vi "AngularCalib.vi"(7 "B [T]":dbl, 10 "Clibration":T13={"cam 0"={"incident ANGLE COMPENSATION"=[], "dp/B [MeV/C/B]"=[], "charge compensation"=[], "Momentum [MeV/C]"=[], "energyDependence Input"=[], "pixel angle (y)"=[], "dp [MeV/C/] "=[], "angle 2Dfor spectrumj"=[], "dp [MeV/C] 2D"=[], "charge compensation 2D"=[], "Screen&Camera 2"={"Screen Orientation"="Regular", "Screen angle"="Flat", "Lens"=enum."FL1-f8x08", "Calibration (mm/pix)"=1.0}, "ROI info"={"npix-X"=0, "npix-Y"=0, "Left [pix]"=0.0, "Top [pix]"=0.0}, "Y 2D full angle"=[], "calib pixel"={"y1(pixel)"=[], "y2(pixel)"=[], "dp/B [MeV/C/B] (pixel)"=[], "energyDependence Input(pixel)"=[], "bending angle [deg](pixel)"=[], "total path(pixel)"=[], "pixel angle (y)(pixel)"=[], "energy dependence (pixel)"=[], "charge compensation (pixel)"=[], "Momentum [MeV/C](pixel)"=[], "angular compensation(pixel)"=[]}, "2D"={"dp"=[], "chargeCompensation"=[], "angle"=[], "Momentum"=[]}, "UserROI"={"Width"=0.0, "Hight"=0.0, "OffsetX"=0.0, "OffsetY"=0.0}, "final"={"X"=[], "xi"=[], "delta momentum"=0.0, "Y"=[], "yi"=[], "angle (Y)"=[], "delta angle"=0.0, "scale delta angle"=0.0, "intraX"=0.0, "intraY"=0.0, "mask"=[]}, "B[T]"=0.0, "index"=0.0}, "cam 1"={"incident ANGLE COMPENSATION"=[], "dp/B [MeV/C/B]"=[], "charge compensation"=[], "Momentum [MeV/C]"=[], "energyDependence Input"=[], "pixel angle (y)"=[], "dp [MeV/C/] "=[], "angle 2Dfor spectrumj"=[], "dp [MeV/C] 2D"=[], "charge compensation 2D"=[], "Screen&Camera 2"={"Screen Orientation"="Regular", "Screen angle"="Flat", "Lens"=enum."FL1-f8x08", "Calibration (mm/pix)"=1.0}, "ROI info"={"npix-X"=0, "npix-Y"=0, "Left [pix]"=0.0, "Top [pix]"=0.0}, "Y 2D full angle"=[], "calib pixel"={"y1(pixel)"=[], "y2(pixel)"=[], "dp/B [MeV/C/B] (pixel)"=[], "energyDependence Input(pixel)"=[], "bending angle [deg](pixel)"=[], "total path(pixel)"=[], "pixel angle (y)(pixel)"=[], "energy dependence (pixel)"=[], "charge compensation (pixel)"=[], "Momentum [MeV/C](pixel)"=[], "angular compensation(pixel)"=[]}, "2D"={"dp"=[], "chargeCompensation"=[], "angle"=[], "Momentum"=[]}, "UserROI"={"Width"=0.0, "Hight"=0.0, "OffsetX"=0.0, "OffsetY"=0.0}, "final"={"X"=[], "xi"=[], "delta momentum"=0.0, "Y"=[], "yi"=[], "angle (Y)"=[], "delta angle"=0.0, "scale delta angle"=0.0, "intraX"=0.0, "intraY"=0.0, "mask"=[]}, "B[T]"=0.0, "index"=0.0}, "cam 2"={"incident ANGLE COMPENSATION"=[], "dp/B [MeV/C/B]"=[], "charge compensation"=[], "Momentum [MeV/C]"=[], "energyDependence Input"=[], "pixel angle (y)"=[], "dp [MeV/C/] "=[], "angle 2Dfor spectrumj"=[], "dp [MeV/C] 2D"=[], "charge compensation 2D"=[], "Screen&Camera 2"={"Screen Orientation"="Regular", "Screen angle"="Flat", "Lens"=enum."FL1-f8x08", "Calibration (mm/pix)"=1.0}, "ROI info"={"npix-X"=0, "npix-Y"=0, "Left [pix]"=0.0, "Top [pix]"=0.0}, "Y 2D full angle"=[], "calib pixel"={"y1(pixel)"=[], "y2(pixel)"=[], "dp/B [MeV/C/B] (pixel)"=[], "energyDependence Input(pixel)"=[], "bending angle [deg](pixel)"=[], "total path(pixel)"=[], "pixel angle (y)(pixel)"=[], "energy dependence (pixel)"=[], "charge compensation (pixel)"=[], "Momentum [MeV/C](pixel)"=[], "angular compensation(pixel)"=[]}, "2D"={"dp"=[], "chargeCompensation"=[], "angle"=[], "Momentum"=[]}, "UserROI"={"Width"=0.0, "Hight"=0.0, "OffsetX"=0.0, "OffsetY"=0.0}, "final"={"X"=[], "xi"=[], "delta momentum"=0.0, "Y"=[], "yi"=[], "angle (Y)"=[], "delta angle"=0.0, "scale delta angle"=0.0, "intraX"=0.0, "intraY"=0.0, "mask"=[]}, "B[T]"=0.0, "index"=0.0}, "cam 3"={"incident ANGLE COMPENSATION"=[], "dp/B [MeV/C/B]"=[], "charge compensation"=[], "Momentum [MeV/C]"=[], "energyDependence Input"=[], "pixel angle (y)"=[], "dp [MeV/C/] "=[], "angle 2Dfor spectrumj"=[], "dp [MeV/C] 2D"=[], "charge compensation 2D"=[], "Screen&Camera 2"={"Screen Orientation"="Regular", "Screen angle"="Flat", "Lens"=enum."FL1-f8x08", "Calibration (mm/pix)"=1.0}, "ROI info"={"npix-X"=0, "npix-Y"=0, "Left [pix]"=0.0, "Top [pix]"=0.0}, "Y 2D full angle"=[], "calib pixel"={"y1(pixel)"=[], "y2(pixel)"=[], "dp/B [MeV/C/B] (pixel)"=[], "energyDependence Input(pixel)"=[], "bending angle [deg](pixel)"=[], "total path(pixel)"=[], "pixel angle (y)(pixel)"=[], "energy dependence (pixel)"=[], "charge compensation (pixel)"=[], "Momentum [MeV/C](pixel)"=[], "angular compensation(pixel)"=[]}, "2D"={"dp"=[], "chargeCompensation"=[], "angle"=[], "Momentum"=[]}, "UserROI"={"Width"=0.0, "Hight"=0.0, "OffsetX"=0.0, "OffsetY"=0.0}, "final"={"X"=[], "xi"=[], "delta momentum"=0.0, "Y"=[], "yi"=[], "angle (Y)"=[], "delta angle"=0.0, "scale delta angle"=0.0, "intraX"=0.0, "intraY"=0.0, "mask"=[]}, "B[T]"=0.0, "index"=0.0}}, 11 "Settings":T1={"CamSettings"={"Cam 0"={"position"=0.0, "pixelsize"=0.0, "start"=0.0, "end"=0.0, "center"=0.0, "Lens"=enum."FL1-f8x08", "Forward"=enum."off", "Spec_Calib_file 2"=path "Y:/100TWdata/ESMCalib/datFwd.txt", "map"=path "Y:/100TWdata/ESMCalib/mapFwd.txt", "y size"=0, "UserROI"={"Width"={"Value"=0.0, "Min"=0.0, "Max"=0.0, "StepSize"=0.0, "Tolerance"=0.0, "ValueActual"=0.0}, "Hight"={"Value"=0.0, "Min"=0.0, "Max"=0.0, "StepSize"=0.0, "Tolerance"=0.0, "ValueActual"=0.0}, "OffsetX"={"Value"=0.0, "Min"=0.0, "Max"=0.0, "StepSize"=0.0, "Tolerance"=0.0, "ValueActual"=0.0}, "OffsetY"={"Value"=0.0, "Min"=0.0, "Max"=0.0, "StepSize"=0.0, "Tolerance"=0.0, "ValueActual"=0.0}}, "CamMaxPixel"={"X"=0, "Y"=0}, "CamROI"={"Width"=0.0, "Hight"=0.0, "OffsetX"=0.0, "OffsetY"=0.0}}, "Cam 1"={"position"=0.0, "pixelsize"=0.0, "start"=0.0, "end"=0.0, "center"=0.0, "Lens"=enum."FL1-f8x08", "Forward"=enum."off", "Spec_Calib_file 2"=path "Y:/100TWdata/ESMCalib/datFwd.txt", "map"=path "Y:/100TWdata/ESMCalib/mapFwd.txt", "y size"=0, "UserROI"={"Width"={"Value"=0.0, "Min"=0.0, "Max"=0.0, "StepSize"=0.0, "Tolerance"=0.0, "ValueActual"=0.0}, "Hight"={"Value"=0.0, "Min"=0.0, "Max"=0.0, "StepSize"=0.0, "Tolerance"=0.0, "ValueActual"=0.0}, "OffsetX"={"Value"=0.0, "Min"=0.0, "Max"=0.0, "StepSize"=0.0, "Tolerance"=0.0, "ValueActual"=0.0}, "OffsetY"={"Value"=0.0, "Min"=0.0, "Max"=0.0, "StepSize"=0.0, "Tolerance"=0.0, "ValueActual"=0.0}}, "CamMaxPixel"={"X"=0, "Y"=0}, "CamROI"={"Width"=0.0, "Hight"=0.0, "OffsetX"=0.0, "OffsetY"=0.0}}, "Cam 2"={"position"=0.0, "pixelsize"=0.0, "start"=0.0, "end"=0.0, "center"=0.0, "Lens"=enum."FL1-f8x08", "Forward"=enum."off", "Spec_Calib_file 2"=path "Y:/100TWdata/ESMCalib/datFwd.txt", "map"=path "Y:/100TWdata/ESMCalib/mapFwd.txt", "y size"=0, "UserROI"={"Width"={"Value"=0.0, "Min"=0.0, "Max"=0.0, "StepSize"=0.0, "Tolerance"=0.0, "ValueActual"=0.0}, "Hight"={"Value"=0.0, "Min"=0.0, "Max"=0.0, "StepSize"=0.0, "Tolerance"=0.0, "ValueActual"=0.0}, "OffsetX"={"Value"=0.0, "Min"=0.0, "Max"=0.0, "StepSize"=0.0, "Tolerance"=0.0, "ValueActual"=0.0}, "OffsetY"={"Value"=0.0, "Min"=0.0, "Max"=0.0, "StepSize"=0.0, "Tolerance"=0.0, "ValueActual"=0.0}}, "CamMaxPixel"={"X"=0, "Y"=0}, "CamROI"={"Width"=0.0, "Hight"=0.0, "OffsetX"=0.0, "OffsetY"=0.0}}, "Cam 3"={"position"=0.0, "pixelsize"=0.0, "start"=0.0, "end"=0.0, "center"=0.0, "Lens"=enum."FL1-f8x08", "Forward"=enum."off", "Spec_Calib_file 2"=path "Y:/100TWdata/ESMCalib/datFwd.txt", "map"=path "Y:/100TWdata/ESMCalib/mapFwd.txt", "y size"=0, "UserROI"={"Width"={"Value"=0.0, "Min"=0.0, "Max"=0.0, "StepSize"=0.0, "Tolerance"=0.0, "ValueActual"=0.0}, "Hight"={"Value"=0.0, "Min"=0.0, "Max"=0.0, "StepSize"=0.0, "Tolerance"=0.0, "ValueActual"=0.0}, "OffsetX"={"Value"=0.0, "Min"=0.0, "Max"=0.0, "StepSize"=0.0, "Tolerance"=0.0, "ValueActual"=0.0}, "OffsetY"={"Value"=0.0, "Min"=0.0, "Max"=0.0, "StepSize"=0.0, "Tolerance"=0.0, "ValueActual"=0.0}}, "CamMaxPixel"={"X"=0, "Y"=0}, "CamROI"={"Width"=0.0, "Hight"=0.0, "OffsetX"=0.0, "OffsetY"=0.0}}}, "timeout"={"Value"=0.0, "Min"=0.0, "Max"=0.0, "StepSize"=0.0, "Tolerance"=0.0, "ValueActual"=0.0}, "Screws"={"Cam 0"={"S 0"={"0"=0, "1"=0, "2"=0, "3"=0}, "S 1"={"0"=0, "1"=0, "2"=0, "3"=0}, "S 2"={"0"=0, "1"=0, "2"=0, "3"=0}, "S 3"={"0"=0, "1"=0, "2"=0, "3"=0}, "S 4"={"0"=0, "1"=0, "2"=0, "3"=0}, "S 5"={"0"=0, "1"=0, "2"=0, "3"=0}}, "Cam 1"={"S 0"={"0"=0, "1"=0, "2"=0, "3"=0}, "S 1"={"0"=0, "1"=0, "2"=0, "3"=0}, "S 2"={"0"=0, "1"=0, "2"=0, "3"=0}, "S 3"={"0"=0, "1"=0, "2"=0, "3"=0}, "S 4"={"0"=0, "1"=0, "2"=0, "3"=0}, "S 5"={"0"=0, "1"=0, "2"=0, "3"=0}}, "Cam 2"={"S 0"={"0"=0, "1"=0, "2"=0, "3"=0}, "S 1"={"0"=0, "1"=0, "2"=0, "3"=0}, "S 2"={"0"=0, "1"=0, "2"=0, "3"=0}, "S 3"={"0"=0, "1"=0, "2"=0, "3"=0}, "S 4"={"0"=0, "1"=0, "2"=0, "3"=0}, "S 5"={"0"=0, "1"=0, "2"=0, "3"=0}}, "Cam 3"={"S 0"={"0"=0, "1"=0, "2"=0, "3"=0}, "S 1"={"0"=0, "1"=0, "2"=0, "3"=0}, "S 2"={"0"=0, "1"=0, "2"=0, "3"=0}, "S 3"={"0"=0, "1"=0, "2"=0, "3"=0}, "S 4"={"0"=0, "1"=0, "2"=0, "3"=0}, "S 5"={"0"=0, "1"=0, "2"=0, "3"=0}}}, "number of cam"=0.0, "X size"=0.0, "srewstart"={"Cam 0"=0.0, "Cam 1"=0.0, "Cam 2"=0.0, "Cam 3"=0.0}, "Save"=enum."off", "offset"=0.0, "localsavingpath"=path "", "ROIString"="", "exposure"={"Value"=0.0, "Min"=0.0, "Max"=0.0, "StepSize"=0.0, "Tolerance"=0.0, "ValueActual"=0.0}, "trigger"=enum."off"}) -> (2 "Clibration 2":T13={"cam 0"={"incident ANGLE COMPENSATION"=[], "dp/B [MeV/C/B]"=[], "charge compensation"=[], "Momentum [MeV/C]"=[], "energyDependence Input"=[], "pixel angle (y)"=[], "dp [MeV/C/] "=[], "angle 2Dfor spectrumj"=[], "dp [MeV/C] 2D"=[], "charge compensation 2D"=[], "Screen&Camera 2"={"Screen Orientation"="Regular", "Screen angle"="Flat", "Lens"=enum."FL1-f8x08", "Calibration (mm/pix)"=1.0}, "ROI info"={"npix-X"=0, "npix-Y"=0, "Left [pix]"=0.0, "Top [pix]"=0.0}, "Y 2D full angle"=[], "calib pixel"={"y1(pixel)"=[], "y2(pixel)"=[], "dp/B [MeV/C/B] (pixel)"=[], "energyDependence Input(pixel)"=[], "bending angle [deg](pixel)"=[], "total path(pixel)"=[], "pixel angle (y)(pixel)"=[], "energy dependence (pixel)"=[], "charge compensation (pixel)"=[], "Momentum [MeV/C](pixel)"=[], "angular compensation(pixel)"=[]}, "2D"={"dp"=[], "chargeCompensation"=[], "angle"=[], "Momentum"=[]}, "UserROI"={"Width"=0.0, "Hight"=0.0, "OffsetX"=0.0, "OffsetY"=0.0}, "final"={"X"=[], "xi"=[], "delta momentum"=0.0, "Y"=[], "yi"=[], "angle (Y)"=[], "delta angle"=0.0, "scale delta angle"=0.0, "intraX"=0.0, "intraY"=0.0, "mask"=[]}, "B[T]"=0.0, "index"=0.0}, "cam 1"={"incident ANGLE COMPENSATION"=[], "dp/B [MeV/C/B]"=[], "charge compensation"=[], "Momentum [MeV/C]"=[], "energyDependence Input"=[], "pixel angle (y)"=[], "dp [MeV/C/] "=[], "angle 2Dfor spectrumj"=[], "dp [MeV/C] 2D"=[], "charge compensation 2D"=[], "Screen&Camera 2"={"Screen Orientation"="Regular", "Screen angle"="Flat", "Lens"=enum."FL1-f8x08", "Calibration (mm/pix)"=1.0}, "ROI info"={"npix-X"=0, "npix-Y"=0, "Left [pix]"=0.0, "Top [pix]"=0.0}, "Y 2D full angle"=[], "calib pixel"={"y1(pixel)"=[], "y2(pixel)"=[], "dp/B [MeV/C/B] (pixel)"=[], "energyDependence Input(pixel)"=[], "bending angle [deg](pixel)"=[], "total path(pixel)"=[], "pixel angle (y)(pixel)"=[], "energy dependence (pixel)"=[], "charge compensation (pixel)"=[], "Momentum [MeV/C](pixel)"=[], "angular compensation(pixel)"=[]}, "2D"={"dp"=[], "chargeCompensation"=[], "angle"=[], "Momentum"=[]}, "UserROI"={"Width"=0.0, "Hight"=0.0, "OffsetX"=0.0, "OffsetY"=0.0}, "final"={"X"=[], "xi"=[], "delta momentum"=0.0, "Y"=[], "yi"=[], "angle (Y)"=[], "delta angle"=0.0, "scale delta angle"=0.0, "intraX"=0.0, "intraY"=0.0, "mask"=[]}, "B[T]"=0.0, "index"=0.0}, "cam 2"={"incident ANGLE COMPENSATION"=[], "dp/B [MeV/C/B]"=[], "charge compensation"=[], "Momentum [MeV/C]"=[], "energyDependence Input"=[], "pixel angle (y)"=[], "dp [MeV/C/] "=[], "angle 2Dfor spectrumj"=[], "dp [MeV/C] 2D"=[], "charge compensation 2D"=[], "Screen&Camera 2"={"Screen Orientation"="Regular", "Screen angle"="Flat", "Lens"=enum."FL1-f8x08", "Calibration (mm/pix)"=1.0}, "ROI info"={"npix-X"=0, "npix-Y"=0, "Left [pix]"=0.0, "Top [pix]"=0.0}, "Y 2D full angle"=[], "calib pixel"={"y1(pixel)"=[], "y2(pixel)"=[], "dp/B [MeV/C/B] (pixel)"=[], "energyDependence Input(pixel)"=[], "bending angle [deg](pixel)"=[], "total path(pixel)"=[], "pixel angle (y)(pixel)"=[], "energy dependence (pixel)"=[], "charge compensation (pixel)"=[], "Momentum [MeV/C](pixel)"=[], "angular compensation(pixel)"=[]}, "2D"={"dp"=[], "chargeCompensation"=[], "angle"=[], "Momentum"=[]}, "UserROI"={"Width"=0.0, "Hight"=0.0, "OffsetX"=0.0, "OffsetY"=0.0}, "final"={"X"=[], "xi"=[], "delta momentum"=0.0, "Y"=[], "yi"=[], "angle (Y)"=[], "delta angle"=0.0, "scale delta angle"=0.0, "intraX"=0.0, "intraY"=0.0, "mask"=[]}, "B[T]"=0.0, "index"=0.0}, "cam 3"={"incident ANGLE COMPENSATION"=[], "dp/B [MeV/C/B]"=[], "charge compensation"=[], "Momentum [MeV/C]"=[], "energyDependence Input"=[], "pixel angle (y)"=[], "dp [MeV/C/] "=[], "angle 2Dfor spectrumj"=[], "dp [MeV/C] 2D"=[], "charge compensation 2D"=[], "Screen&Camera 2"={"Screen Orientation"="Regular", "Screen angle"="Flat", "Lens"=enum."FL1-f8x08", "Calibration (mm/pix)"=1.0}, "ROI info"={"npix-X"=0, "npix-Y"=0, "Left [pix]"=0.0, "Top [pix]"=0.0}, "Y 2D full angle"=[], "calib pixel"={"y1(pixel)"=[], "y2(pixel)"=[], "dp/B [MeV/C/B] (pixel)"=[], "energyDependence Input(pixel)"=[], "bending angle [deg](pixel)"=[], "total path(pixel)"=[], "pixel angle (y)(pixel)"=[], "energy dependence (pixel)"=[], "charge compensation (pixel)"=[], "Momentum [MeV/C](pixel)"=[], "angular compensation(pixel)"=[]}, "2D"={"dp"=[], "chargeCompensation"=[], "angle"=[], "Momentum"=[]}, "UserROI"={"Width"=0.0, "Hight"=0.0, "OffsetX"=0.0, "OffsetY"=0.0}, "final"={"X"=[], "xi"=[], "delta momentum"=0.0, "Y"=[], "yi"=[], "angle (Y)"=[], "delta angle"=0.0, "scale delta angle"=0.0, "intraX"=0.0, "intraY"=0.0, "mask"=[]}, "B[T]"=0.0, "index"=0.0}}, 3 "Settings OUT":T1={"CamSettings"={"Cam 0"={"position"=0.0, "pixelsize"=0.0, "start"=0.0, "end"=0.0, "center"=0.0, "Lens"=enum."FL1-f8x08", "Forward"=enum."off", "Spec_Calib_file 2"=path "Y:/100TWdata/ESMCalib/datFwd.txt", "map"=path "Y:/100TWdata/ESMCalib/mapFwd.txt", "y size"=0, "UserROI"={"Width"={"Value"=0.0, "Min"=0.0, "Max"=0.0, "StepSize"=0.0, "Tolerance"=0.0, "ValueActual"=0.0}, "Hight"={"Value"=0.0, "Min"=0.0, "Max"=0.0, "StepSize"=0.0, "Tolerance"=0.0, "ValueActual"=0.0}, "OffsetX"={"Value"=0.0, "Min"=0.0, "Max"=0.0, "StepSize"=0.0, "Tolerance"=0.0, "ValueActual"=0.0}, "OffsetY"={"Value"=0.0, "Min"=0.0, "Max"=0.0, "StepSize"=0.0, "Tolerance"=0.0, "ValueActual"=0.0}}, "CamMaxPixel"={"X"=0, "Y"=0}, "CamROI"={"Width"=0.0, "Hight"=0.0, "OffsetX"=0.0, "OffsetY"=0.0}}, "Cam 1"={"position"=0.0, "pixelsize"=0.0, "start"=0.0, "end"=0.0, "center"=0.0, "Lens"=enum."FL1-f8x08", "Forward"=enum."off", "Spec_Calib_file 2"=path "Y:/100TWdata/ESMCalib/datFwd.txt", "map"=path "Y:/100TWdata/ESMCalib/mapFwd.txt", "y size"=0, "UserROI"={"Width"={"Value"=0.0, "Min"=0.0, "Max"=0.0, "StepSize"=0.0, "Tolerance"=0.0, "ValueActual"=0.0}, "Hight"={"Value"=0.0, "Min"=0.0, "Max"=0.0, "StepSize"=0.0, "Tolerance"=0.0, "ValueActual"=0.0}, "OffsetX"={"Value"=0.0, "Min"=0.0, "Max"=0.0, "StepSize"=0.0, "Tolerance"=0.0, "ValueActual"=0.0}, "OffsetY"={"Value"=0.0, "Min"=0.0, "Max"=0.0, "StepSize"=0.0, "Tolerance"=0.0, "ValueActual"=0.0}}, "CamMaxPixel"={"X"=0, "Y"=0}, "CamROI"={"Width"=0.0, "Hight"=0.0, "OffsetX"=0.0, "OffsetY"=0.0}}, "Cam 2"={"position"=0.0, "pixelsize"=0.0, "start"=0.0, "end"=0.0, "center"=0.0, "Lens"=enum."FL1-f8x08", "Forward"=enum."off", "Spec_Calib_file 2"=path "Y:/100TWdata/ESMCalib/datFwd.txt", "map"=path "Y:/100TWdata/ESMCalib/mapFwd.txt", "y size"=0, "UserROI"={"Width"={"Value"=0.0, "Min"=0.0, "Max"=0.0, "StepSize"=0.0, "Tolerance"=0.0, "ValueActual"=0.0}, "Hight"={"Value"=0.0, "Min"=0.0, "Max"=0.0, "StepSize"=0.0, "Tolerance"=0.0, "ValueActual"=0.0}, "OffsetX"={"Value"=0.0, "Min"=0.0, "Max"=0.0, "StepSize"=0.0, "Tolerance"=0.0, "ValueActual"=0.0}, "OffsetY"={"Value"=0.0, "Min"=0.0, "Max"=0.0, "StepSize"=0.0, "Tolerance"=0.0, "ValueActual"=0.0}}, "CamMaxPixel"={"X"=0, "Y"=0}, "CamROI"={"Width"=0.0, "Hight"=0.0, "OffsetX"=0.0, "OffsetY"=0.0}}, "Cam 3"={"position"=0.0, "pixelsize"=0.0, "start"=0.0, "end"=0.0, "center"=0.0, "Lens"=enum."FL1-f8x08", "Forward"=enum."off", "Spec_Calib_file 2"=path "Y:/100TWdata/ESMCalib/datFwd.txt", "map"=path "Y:/100TWdata/ESMCalib/mapFwd.txt", "y size"=0, "UserROI"={"Width"={"Value"=0.0, "Min"=0.0, "Max"=0.0, "StepSize"=0.0, "Tolerance"=0.0, "ValueActual"=0.0}, "Hight"={"Value"=0.0, "Min"=0.0, "Max"=0.0, "StepSize"=0.0, "Tolerance"=0.0, "ValueActual"=0.0}, "OffsetX"={"Value"=0.0, "Min"=0.0, "Max"=0.0, "StepSize"=0.0, "Tolerance"=0.0, "ValueActual"=0.0}, "OffsetY"={"Value"=0.0, "Min"=0.0, "Max"=0.0, "StepSize"=0.0, "Tolerance"=0.0, "ValueActual"=0.0}}, "CamMaxPixel"={"X"=0, "Y"=0}, "CamROI"={"Width"=0.0, "Hight"=0.0, "OffsetX"=0.0, "OffsetY"=0.0}}}, "timeout"={"Value"=0.0, "Min"=0.0, "Max"=0.0, "StepSize"=0.0, "Tolerance"=0.0, "ValueActual"=0.0}, "Screws"={"Cam 0"={"S 0"={"0"=0, "1"=0, "2"=0, "3"=0}, "S 1"={"0"=0, "1"=0, "2"=0, "3"=0}, "S 2"={"0"=0, "1"=0, "2"=0, "3"=0}, "S 3"={"0"=0, "1"=0, "2"=0, "3"=0}, "S 4"={"0"=0, "1"=0, "2"=0, "3"=0}, "S 5"={"0"=0, "1"=0, "2"=0, "3"=0}}, "Cam 1"={"S 0"={"0"=0, "1"=0, "2"=0, "3"=0}, "S 1"={"0"=0, "1"=0, "2"=0, "3"=0}, "S 2"={"0"=0, "1"=0, "2"=0, "3"=0}, "S 3"={"0"=0, "1"=0, "2"=0, "3"=0}, "S 4"={"0"=0, "1"=0, "2"=0, "3"=0}, "S 5"={"0"=0, "1"=0, "2"=0, "3"=0}}, "Cam 2"={"S 0"={"0"=0, "1"=0, "2"=0, "3"=0}, "S 1"={"0"=0, "1"=0, "2"=0, "3"=0}, "S 2"={"0"=0, "1"=0, "2"=0, "3"=0}, "S 3"={"0"=0, "1"=0, "2"=0, "3"=0}, "S 4"={"0"=0, "1"=0, "2"=0, "3"=0}, "S 5"={"0"=0, "1"=0, "2"=0, "3"=0}}, "Cam 3"={"S 0"={"0"=0, "1"=0, "2"=0, "3"=0}, "S 1"={"0"=0, "1"=0, "2"=0, "3"=0}, "S 2"={"0"=0, "1"=0, "2"=0, "3"=0}, "S 3"={"0"=0, "1"=0, "2"=0, "3"=0}, "S 4"={"0"=0, "1"=0, "2"=0, "3"=0}, "S 5"={"0"=0, "1"=0, "2"=0, "3"=0}}}, "number of cam"=0.0, "X size"=0.0, "srewstart"={"Cam 0"=0.0, "Cam 1"=0.0, "Cam 2"=0.0, "Cam 3"=0.0}, "Save"=enum."off", "offset"=0.0, "localsavingpath"=path "", "ROIString"="", "exposure"={"Value"=0.0, "Min"=0.0, "Max"=0.0, "StepSize"=0.0, "Tolerance"=0.0, "ValueActual"=0.0}, "trigger"=enum."off"})   [LabVIEW 2013]
uses:
  Calib_Typdef.ctl
  calib_Sub_Typdef.ctl
  ScreenCam2_TypDEf.ctl
  MagAnalysis_Online_Bella/SubVis/CamAndObj_TypDEf.ctl
  ROIInfo_TypDef.ctl
  calibPixel.ctl
  2DTypDef.ctl
  CamRoiTypDef.ctl
  finalCalibTypdef.ctl
  settings_TypDef.ctl
  CamSettings_Typdef.ctl
  CamSettingSUB_TypDEf.ctl
  shared/OnOffTypeDef.ctl
  userROI.ctl
  shared/numericVariable_TypeDef.ctl
  SrewMaster_TYpDef.ctl
  srew_TypDEf.ctl
  ScrewSub_Typdef.ctl
  screwstart.ctl
  BaseDriver/BaseDriver.lvclass
  MagAnalysis_Online.lvclass
panel:
  out "error in (no error)":errorcluster
  out "number of cam":dbl
  out "Numeric":i32
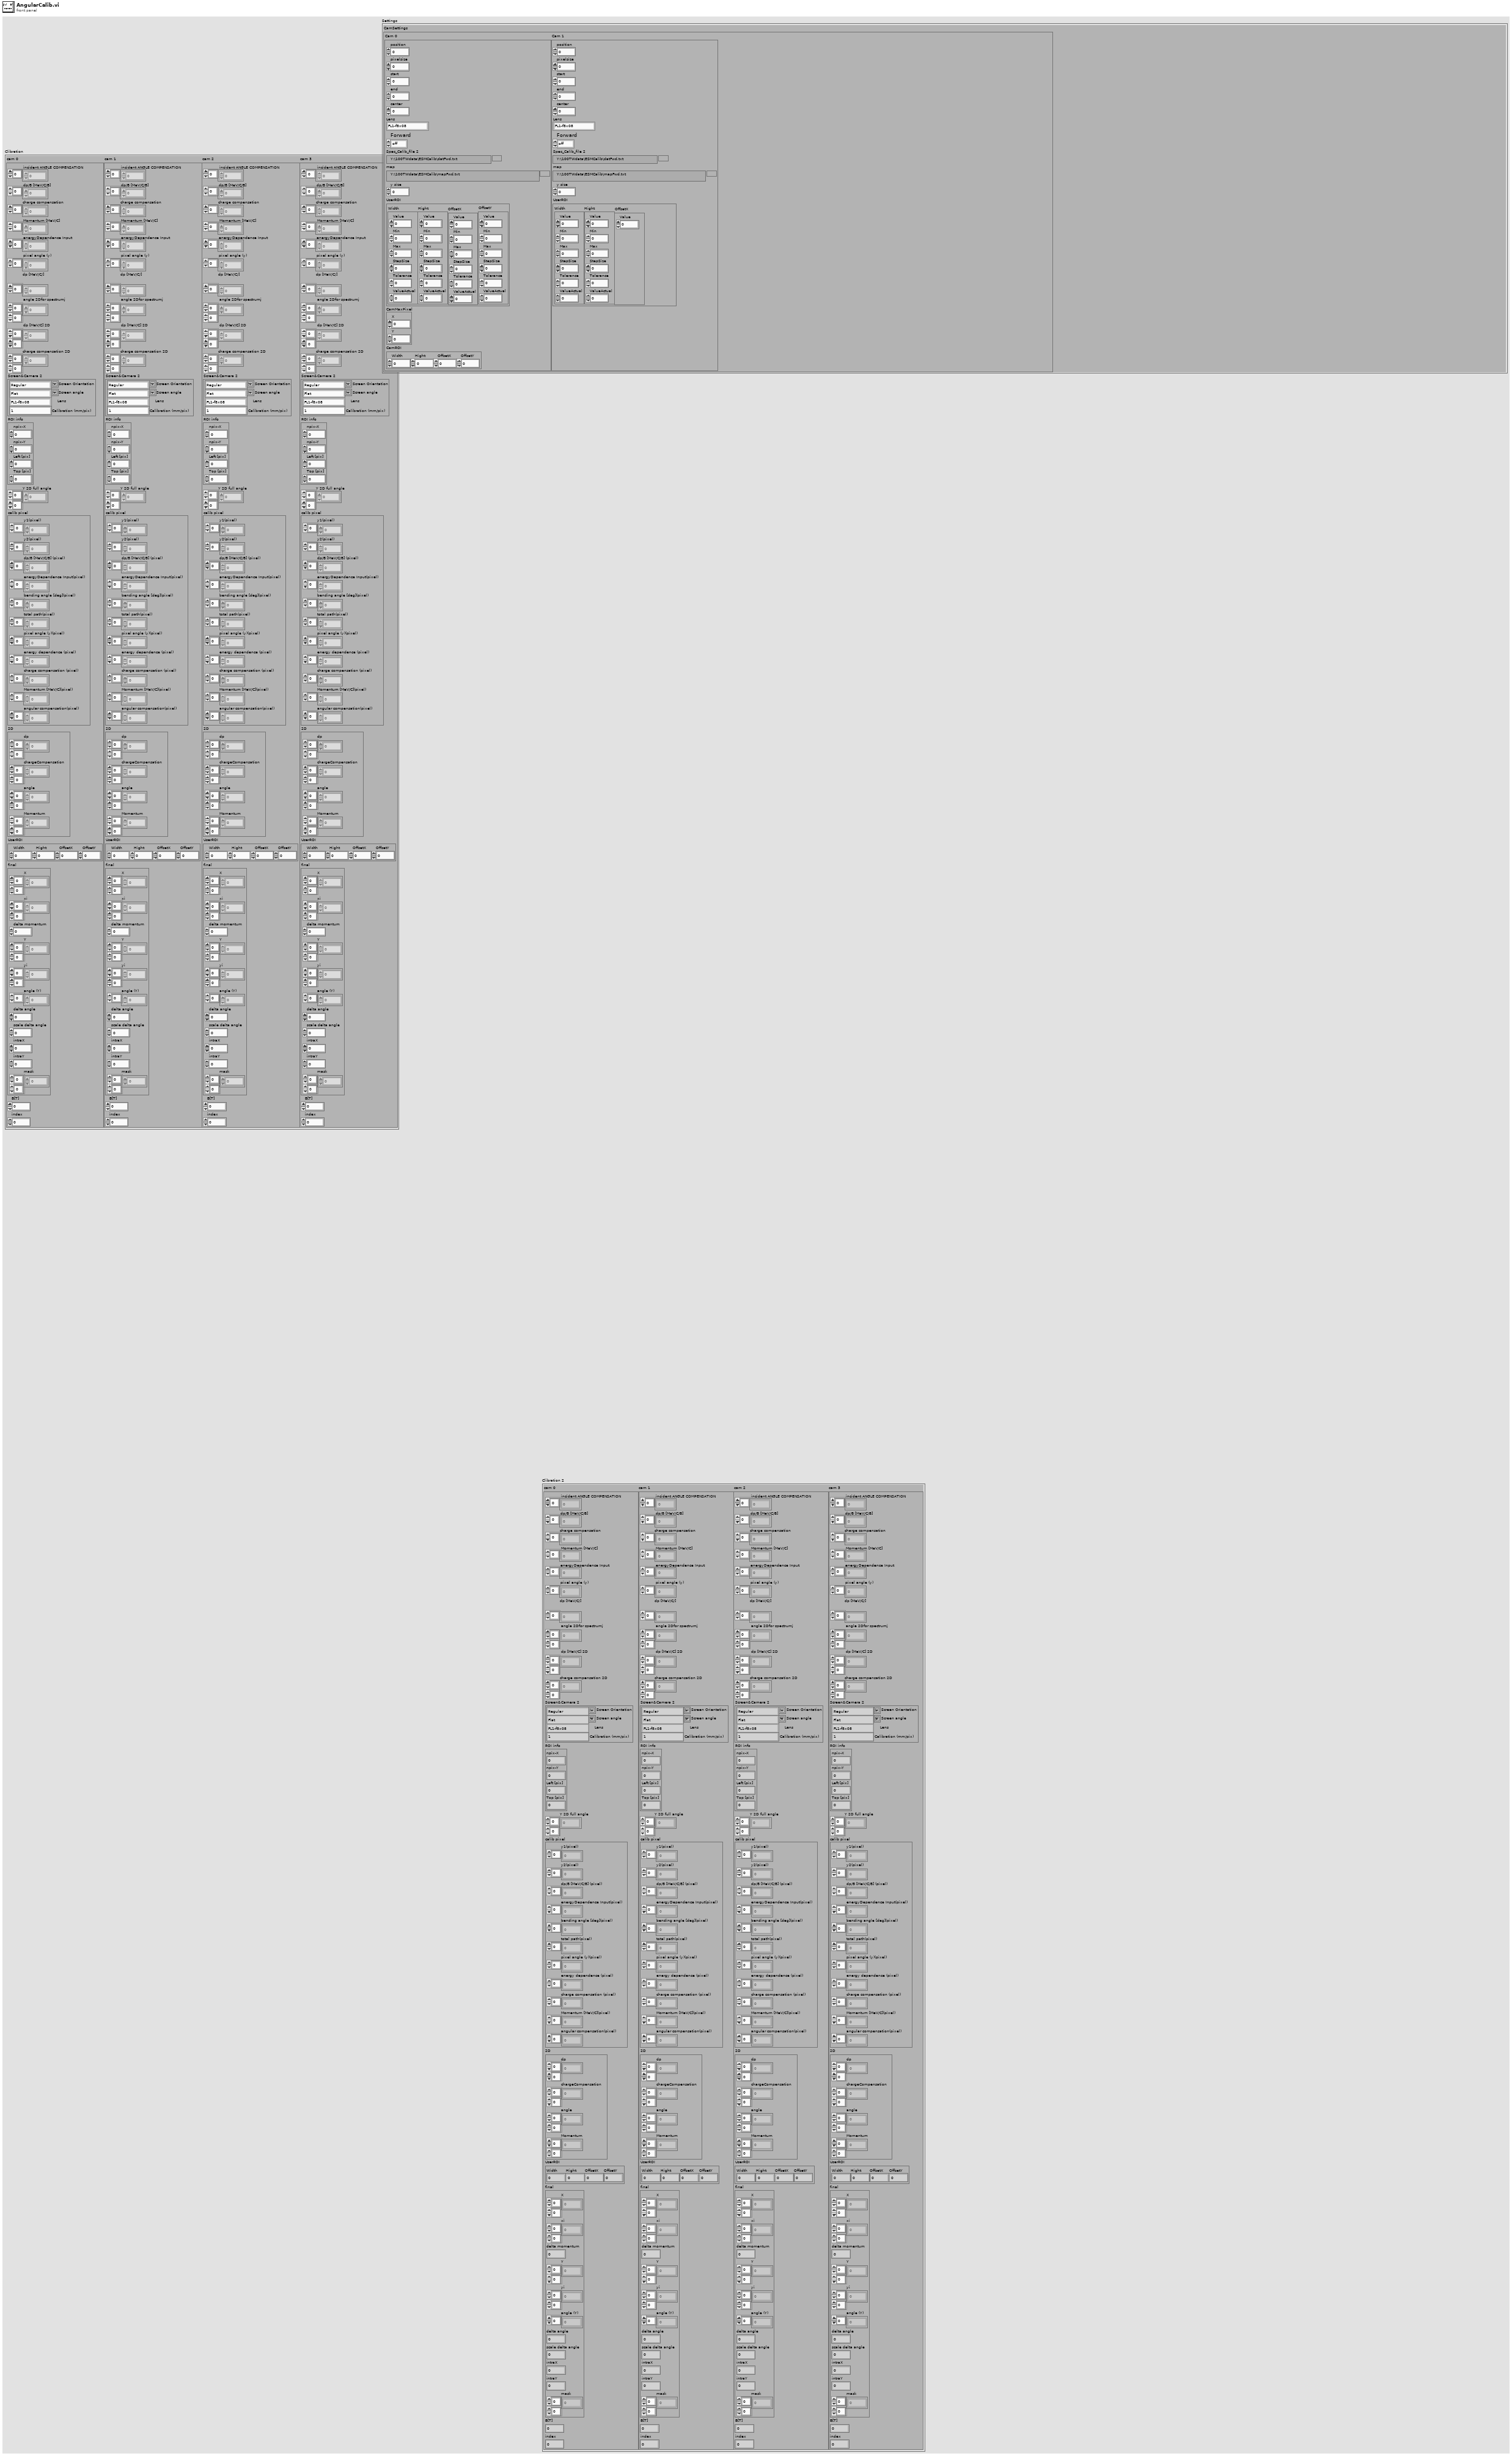
[diagram p1: front panel]
types:
  T1 = typedef "MagAnalysis_Online.lvclass/settings_TypDef.ctl" = cluster{"CamSettings":T2, "timeout":T7, "Screws":T9, "number of cam":dbl, "X size":dbl, "srewstart":T12, "Save":T5, "offset":dbl, "localsavingpath":path, "ROIString":string, "exposure":T7, "trigger":T5}
  T2 = typedef "CamSettings_Typdef.ctl" = cluster{"Cam 0":T3, "Cam 1":T3, "Cam 2":T3, "Cam 3":T3}
  T3 = typedef "CamSettingSUB_TypDEf.ctl" = cluster{"position":dbl, "pixelsize":dbl, "start":dbl, "end":dbl, "center":dbl, "Lens":T4, "Forward":T5, "Spec_Calib_file 2":path, "map":path, "y size":i32, "UserROI":T6, "CamMaxPixel":cluster{"X":i32, "Y":i32}, "CamROI":T8}
  T4 = typedef "CamAndObj_TypDEf.ctl" = enum16{"FL1-f8x08", "FL1-f8x06", "FL1-f8", "ch300-f50", "FL2G-f8", "FL3M14-f8", "FL3M14-f8x08", "FL3M14-f8x08(2x2)"}
  T5 = typedef "OnOffTypeDef.ctl" = enum16{"off", "on"}
  T6 = typedef "userROI.ctl" = cluster{"Width":T7, "Hight":T7, "OffsetX":T7, "OffsetY":T7}
  T7 = typedef "BaseDriver.lvclass/numericVariable_TypeDef.ctl" = cluster{"Value":dbl, "Min":dbl, "Max":dbl, "StepSize":dbl, "Tolerance":dbl, "ValueActual":dbl}
  T8 = typedef "CamRoiTypDef.ctl" = cluster{"Width":dbl, "Hight":dbl, "OffsetX":dbl, "OffsetY":dbl}
  T9 = typedef "SrewMaster_TYpDef.ctl" = cluster{"Cam 0":T10, "Cam 1":T10, "Cam 2":T10, "Cam 3":T10}
  T10 = typedef "srew_TypDEf.ctl" = cluster{"S 0":T11, "S 1":T11, "S 2":T11, "S 3":T11, "S 4":T11, "S 5":T11}
  T11 = typedef "ScrewSub_Typdef.ctl" = cluster{"0":i32, "1":i32, "2":i32, "3":i32}
  T12 = typedef "screwstart.ctl" = cluster{"Cam 0":dbl, "Cam 1":dbl, "Cam 2":dbl, "Cam 3":dbl}
  T13 = typedef "Calib_Typdef.ctl" = cluster{"cam 0":T14, "cam 1":T14, "cam 2":T14, "cam 3":T14}
  T14 = typedef "calib_Sub_Typdef.ctl" = cluster{"incident ANGLE COMPENSATION":dbl[], "dp/B [MeV/C/B]":dbl[], "charge compensation":dbl[], "Momentum [MeV/C]":dbl[], "energyDependence Input":dbl[], "pixel angle (y)":dbl[], "dp [MeV/C/] ":dbl[], "angle 2Dfor spectrumj":dbl[][], "dp [MeV/C] 2D":dbl[][], "charge compensation 2D":dbl[][], "Screen&Camera 2":T15, "ROI info":T16, "Y 2D full angle":dbl[][], "calib pixel":T17, "2D":T18, "UserROI":T8, "final":T19, "B[T]":dbl, "index":dbl}
  T15 = typedef "ScreenCam2_TypDEf.ctl" = cluster{"Screen Orientation":string, "Screen angle":string, "Lens":T4, "Calibration (mm/pix)":dbl}
  T16 = typedef "ROIInfo_TypDef.ctl" = cluster{"npix-X":i32, "npix-Y":i32, "Left [pix]":dbl, "Top [pix]":dbl}
  T17 = typedef "calibPixel.ctl" = cluster{"y1(pixel)":dbl[], "y2(pixel)":dbl[], "dp/B [MeV/C/B] (pixel)":dbl[], "energyDependence Input(pixel)":dbl[], "bending angle [deg](pixel)":dbl[], "total path(pixel)":dbl[], "pixel angle (y)(pixel)":dbl[], "energy dependence (pixel)":dbl[], "charge compensation (pixel)":dbl[], "Momentum [MeV/C](pixel)":dbl[], "angular compensation(pixel)":dbl[]}
  T18 = typedef "2DTypDef.ctl" = cluster{"dp":dbl[][], "chargeCompensation":dbl[][], "angle":dbl[][], "Momentum":dbl[][]}
  T19 = typedef "finalCalibTypdef.ctl" = cluster{"X":dbl[][], "xi":dbl[][], "delta momentum":dbl, "Y":dbl[][], "yi":dbl[][], "angle (Y)":dbl[], "delta angle":dbl, "scale delta angle":dbl, "intraX":dbl, "intraY":dbl, "mask":dbl[][]}
  T20 = cluster{"[0]":T14, "[1]":T14, "[2]":T14, "[3]":T14}
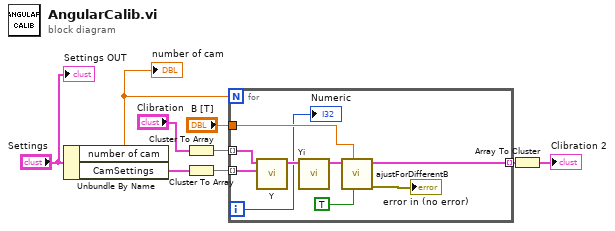
[diagram p0: block diagram]
diagram:
  n1 = Unbundle By Name("Settings") -> ("number of cam"=w1:dbl, "CamSettings"=w3:T2)
  "number of cam" <- w1
  n2 = Cluster To Array(cluster="Clibration") -> (array=w6:T14[])
  n3 = Cluster To Array(cluster=w3) -> (array=w7:T3[])
  n4 = for {
    N: w1 -> [_]
    tunnel: w6 -> [w17] mode=indexing
    tunnel: w7 -> [w18] mode=indexing
    tunnel: [w14] -> w8 mode=indexing
    tunnel: "B [T]" -> [w13]
    i -> [w11]
    n5 = call "Y.vi"("Cam 0"=w18, "cam 0"=w17) -> ("cam out"=w16:T14)  [unwired: 9 in]
    n6 = call "Yi.vi"("cam 0"=w16) -> ("output cluster"=w15:T14)  [unwired: 9 in, 1 out]
    n7 = call "ajustForDifferentB.vi"("force (FALSE)"=TRUE, "B [T]"=w13, "Cam Cluster out in"=w15) -> ("error in (no error)"=→"error in (no error)":errorcluster, "Cam Cluster out out"=w14:T14)  [unwired: 7 in]
    "Numeric" <- w11
  }
  n8 = Array To Cluster(array=w8) -> (cluster=→"Clibration 2":T20)
  "Settings OUT" <- "Settings"
